vi "ThreeIncoming_ThreeDataTypes_Bitpacked.vi"() -> ()   [LabVIEW 2019]
uses:
  <vilib>/rvi/DataTransferAndStorage/Container/XNode/niFpgaContainer.xnode
  <vilib>/rvi/interface/RandomDataEmulation/nirviRandomDataFpgaReadWriteTemplate.vi
panel:
  in  "FXP27.5":fxp<+/-,27,5>
  out "FXP27.5 out":fxp<+/-,27,5>
  in  "FXP20.5":fxp<+/-,20,5>
  out "FXP20.5 out":fxp<+/-,20,5>
  in  "FXP16.7":fxp<+/-,16,7>
  out "FXP16.7 out":fxp<+/-,16,7>
  out "FXP64.32 out":fxp<+/-,64,32>
  out "FXP32.8 out":fxp<+/-,32,8>
  out "FXP16.5 out":fxp<+/-,16,5>
  out "FXP24.5 out":fxp<+/-,24,5>
  in  "FXP64.32":fxp<+/-,64,32>
  in  "FXP32.8":fxp<+/-,32,8>
  in  "FXP16.5":fxp<+/-,16,5>
  in  "FXP24.5":fxp<+/-,24,5>
  out "Boolean 2":bool=TRUE
  out "Fast timeout":bool
  out "Med timeout":bool
  out "Slow timeout":bool
  in  "I16":i16
  in  "I8":i8
  in  "I64":i64
  in  "I32":i32
  in  "U16":u16
  in  "U8":u8
  in  "U64":u64
  in  "U32":u32
  in  "SGL":sgl
  in  "Boolean":bool
  out "I16 out":i16
  out "I8 out":i8
  out "I64 out":i64
  out "I32 out":i32
  out "U16 out":u16
  out "U8 out":u8
  out "U64 out":u64
  out "U32 out":u32
  out "SGL out":sgl
  out "Boolean out":bool
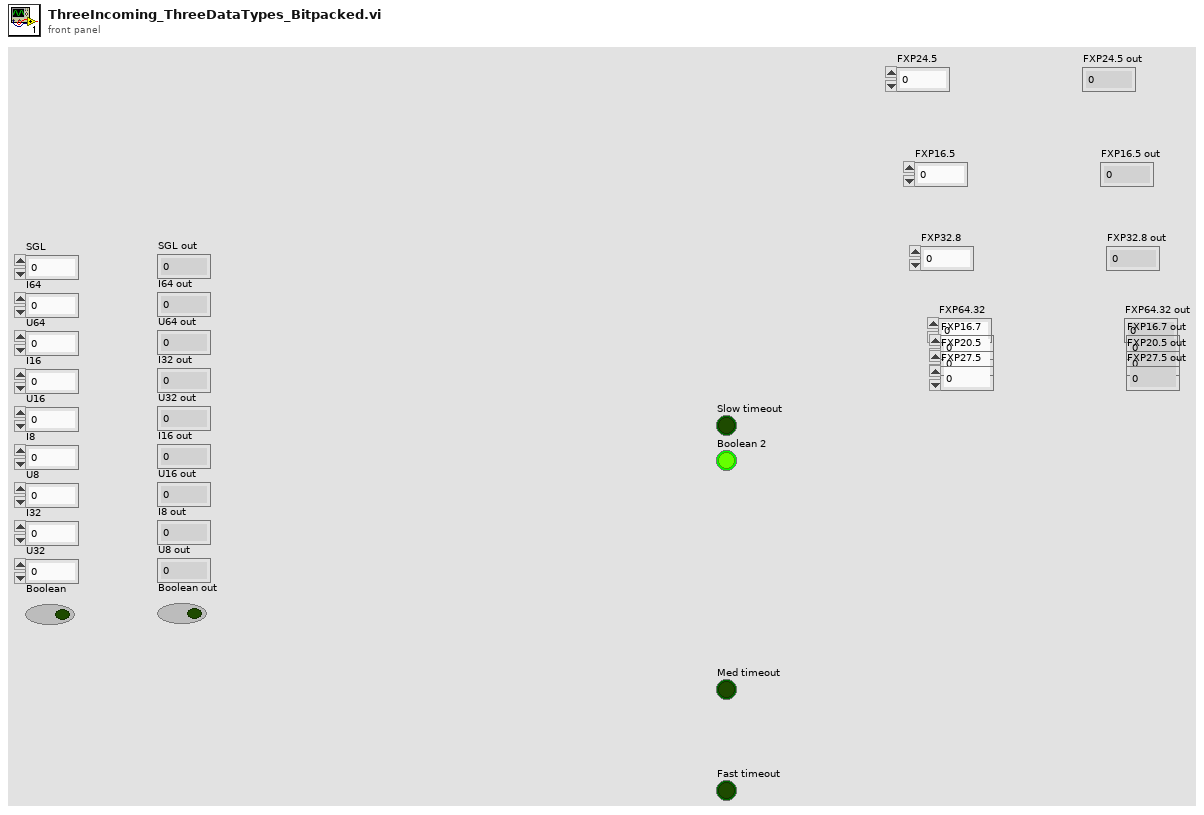
[diagram p1: front panel]
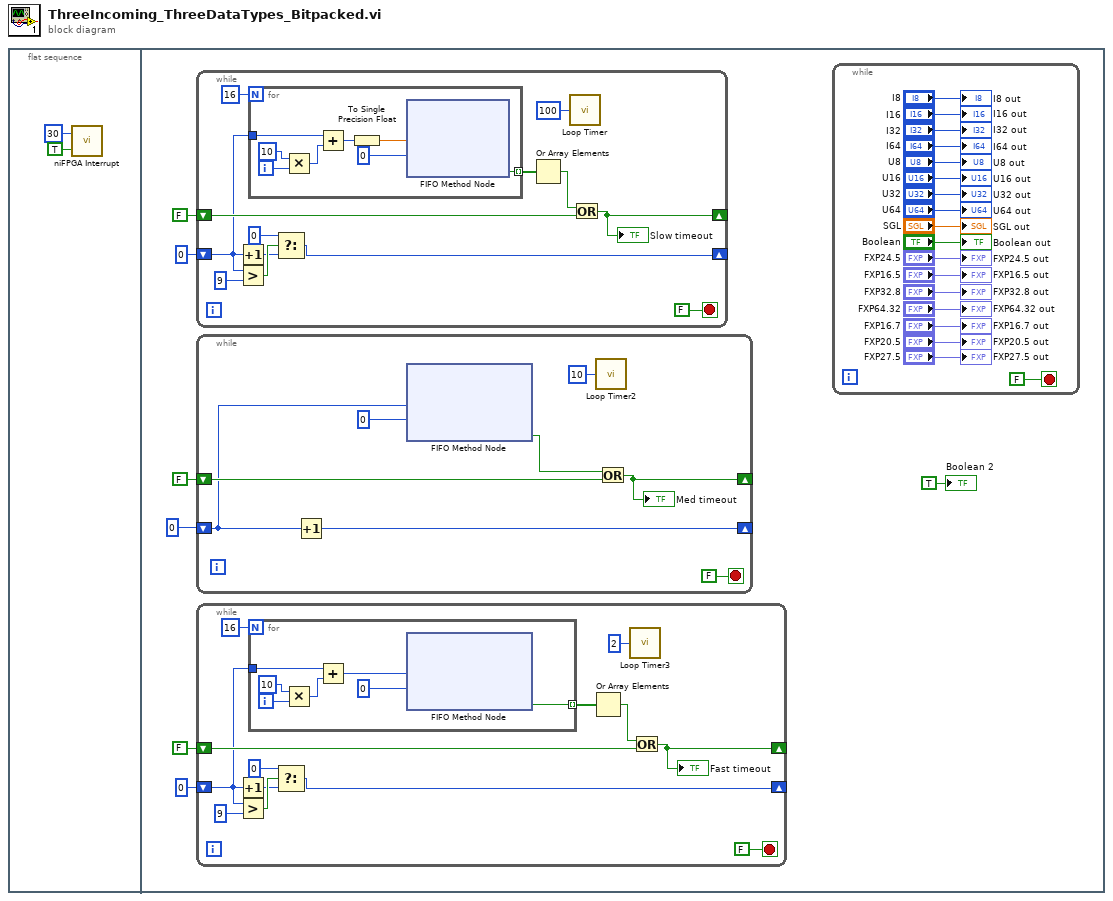
[diagram p0: block diagram]
diagram:
  n1 = flat-sequence {
    frame #0 {
      n2 = call <vilib>:"niFPGA Interrupt.vi"("Wait Until Cleared (F)"=TRUE, "IRQ Number (0)"=u8 30) -> ()  [unwired: 1 in]
    }
    frame #1 {
      n3 = while {
        shift-right: [w45] -> _
        shift-left: 0 ("t") -> [w38]
        shift-right: [w39] -> _
        shift-left: FALSE -> [w40]
        stop <- FALSE stop-if-true
        n4 = Increment(x=w38) -> (x+1=w43:i32)
        n5 = Greater?(x=w38, y=9) -> (0:w49:bool)
        n6 = for {
          N: 16 -> [_]
          tunnel: w38 -> [w58]
          tunnel: [w51] -> w42 mode=indexing
          i -> [w57]
          n7 = Multiply(x=10, y=w57) -> (x*y=w55:i32)
          n8 = Add(x=w58, y=w55) -> (x+y=w54:i32)
          n9 = To Single Precision Float(number=w54) -> (single precision float=w53:sgl)
          n10 = xnode ("FIFO Method Node")("Element"=w53, "Timeout"=0) -> ("Timed Out?"=w51:bool)  [unwired: 1 in, 1 out]
        }
        n11 = Select(t=0, s=w49, f=w43) -> (s? t:f=w45:i32)
        n12 = Or Array Elements(Boolean array=w42) -> (logical OR=w41:bool)
        n13 = call "Loop Timer"("Count(uSec)"=u32 100) -> ()  [unwired: 1 out]
        n14 = Or(x=w41, y=w40) -> (x .or. y?=w39:bool)
        "Slow timeout" <- w39
      }
      n15 = while {
        shift-right: [w34] -> _
        shift-left: FALSE -> [w35]
        shift-right: [w30] -> _
        shift-left: u64 0 -> [w31]
        stop <- FALSE stop-if-true
        n16 = Increment(x=w31) -> (x+1=w30:u64)
        n17 = xnode ("FIFO Method Node")("Element"=w31, "Timeout"=0) -> ("Timed Out?"=w32:bool)  [unwired: 1 in, 1 out]
        n18 = call "Loop Timer2"("Count(uSec)"=u32 10) -> ()  [unwired: 1 out]
        n19 = Or(x=w32, y=w35) -> (x .or. y?=w34:bool)
        "Med timeout" <- w34
      }
      n20 = while {
        shift-right: [w17] -> _
        shift-left: 0 ("t") -> [w10]
        shift-right: [w11] -> _
        shift-left: FALSE -> [w12]
        stop <- FALSE stop-if-true
        n21 = Increment(x=w10) -> (x+1=w15:i32)
        n22 = Greater?(x=w10, y=9) -> (0:w21:bool)
        n23 = for {
          N: 16 -> [_]
          tunnel: w10 -> [w29]
          tunnel: [w24] -> w14 mode=indexing
          i -> [w28]
          n24 = Multiply(x=10, y=w28) -> (x*y=w26:i32)
          n25 = Add(x=w29, y=w26) -> (x+y=w23:i32)
          n26 = xnode ("FIFO Method Node")("Element"=w23, "Timeout"=0) -> ("Timed Out?"=w24:bool)  [unwired: 1 in, 1 out]
        }
        n27 = Select(t=0, s=w21, f=w15) -> (s? t:f=w17:i32)
        n28 = Or Array Elements(Boolean array=w14) -> (logical OR=w13:bool)
        n29 = call "Loop Timer3"("Count(uSec)"=u32 2) -> ()  [unwired: 1 out]
        n30 = Or(x=w13, y=w12) -> (x .or. y?=w11:bool)
        "Fast timeout" <- w11
      }
      n31 = while {
        stop <- FALSE stop-if-true
        "I16 out" <- "I16"
        "I8 out" <- "I8"
        "I64 out" <- "I64"
        "I32 out" <- "I32"
        "U16 out" <- "U16"
        "U8 out" <- "U8"
        "U64 out" <- "U64"
        "U32 out" <- "U32"
        "SGL out" <- "SGL"
        "Boolean out" <- "Boolean"
        "FXP24.5 out" <- "FXP24.5"
        "FXP16.5 out" <- "FXP16.5"
        "FXP32.8 out" <- "FXP32.8"
        "FXP64.32 out" <- "FXP64.32"
        "FXP16.7 out" <- "FXP16.7"
        "FXP20.5 out" <- "FXP20.5"
        "FXP27.5 out" <- "FXP27.5"
      }
      "Boolean 2" <- TRUE
    }
  }
